vi "state_and_args.vi"(9 "String":string, 11 "DELIMITER (:)":string=":") -> (1 "Arguments":string, 2 "State":string)   [LabVIEW 2019]
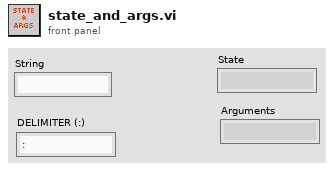
[diagram p1: front panel]
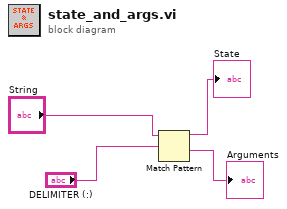
[diagram p0: block diagram]
diagram:
  n1 = Match Pattern(string="String", regular expression="DELIMITER (:)") -> (before substring=→"State":string, after substring=→"Arguments":string)  [unwired: 1 in, 2 out]
